vi "AutoShootTime.vi"(6 "StartTime(ms)":u32, 11 "ShootTime(ms)":u32) -> (3 "Complete":bool)   [LabVIEW 2019]
uses:
  Implements/Shooter/TypeDefs/Hood_Homing_State.ctl
  ArgosLib/Signal Processing/TypeDefs/EdgeDetector_Type.ctl
  Global_Var-RefNum/RobotState.vi
  Global_Var-RefNum/AutoCommands.vi
  ArgosLib/ArgosLib.lvlib
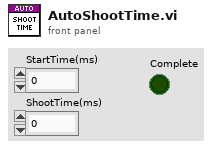
[diagram p1: front panel]
types:
  T1 = typedef "ArgosLib.lvlib/EdgeDetector_Type.ctl" = enum16{"RisingEdge", "FallingEdge", "Both"}
  T2 = typedef "Hood_Homing_State.ctl" = enum16{"Not Homed", "Homing in Process", "Homing Failed", "Homing Completed"}
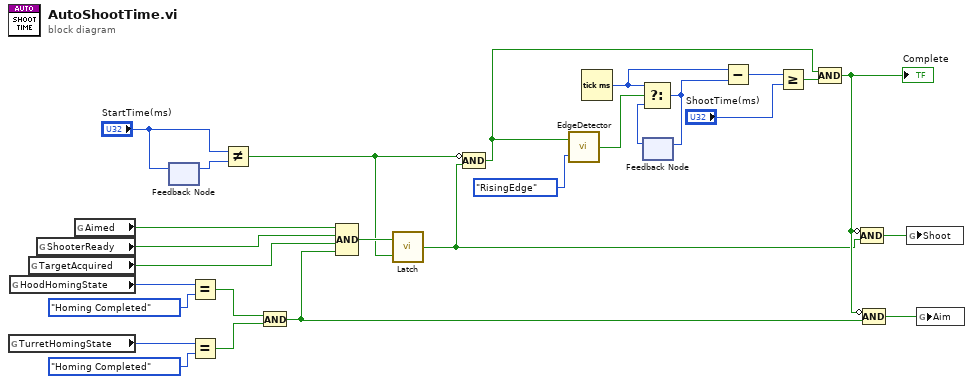
[diagram p0: block diagram]
diagram:
  n1 = global read "RobotState.vi" "TurretHomingState"() -> (w27:T2)
  n2 = global read "RobotState.vi" "HoodHomingState"() -> (w24:T2)
  n3 = global read "RobotState.vi" "TargetAcquired"() -> (w19:bool)
  n4 = global read "RobotState.vi" "ShooterReady"() -> (w20:bool)
  n5 = global read "RobotState.vi" "Aimed"() -> (w21:bool)
  n6 = feedback-in #1("StartTime(ms)") -> ()
  n7 = feedback #1() -> (w18:u32)  [unwired: 1 in]
  n8 = Equal?(x=w24, y=Hood_Homing_State."Homing Completed") -> (x = y?=w23:bool)
  n9 = Equal?(x=w27, y=Hood_Homing_State."Homing Completed") -> (x = y?=w22:bool)
  n10 = Not Equal?(x="StartTime(ms)", y=w18) -> (x != y?=w2:bool)
  n11 = And(x=w23, y=w22) -> (x .and. y?=w9:bool)
  n12 = Compound Arithmetic op=AND(w21, w20, w19, w9) -> (w3:bool)
  n13 = call "Latch.vi"("Reset"=w2, "Input"=w3) -> ("LatchOut"=w1:bool)
  n14 = Compound Arithmetic op=AND(invert w2, w1) -> (w5:bool)
  n15 = call "EdgeDetector.vi"("DetectorType"=EdgeDetector_Type."RisingEdge", "Input"=w5) -> ("Edge"=w15:bool)
  n16 = Tick Count (ms)() -> (millisecond timer value=w13:u32)
  n17 = feedback #2() -> (w14:u32)  [unwired: 1 in]
  n18 = Select(t=w13, s=w15, f=w14) -> (s? t:f=w12:u32)
  n19 = feedback-in #2(w12) -> ()
  n20 = Subtract(x=w13, y=w12) -> (x-y=w11:u32)
  n21 = Greater Or Equal?(x=w11, y="ShootTime(ms)") -> (x >= y?=w6:bool)
  n22 = Compound Arithmetic op=AND(w5, w6) -> (w4:bool)
  "Complete" <- w4
  n23 = Compound Arithmetic op=AND(invert w4, w1) -> (w7:bool)
  n24 = Compound Arithmetic op=AND(invert w4, w9) -> (w8:bool)
  n25 = global write "AutoCommands.vi" "Shoot"(w7) -> ()
  n26 = global write "AutoCommands.vi" "Aim"(w8) -> ()
